vi "MessageCore.vi"(6 "Timeout (ms)":i32=-1, 8 "error in (no error)":errorcluster, 9 "Payload":string, 10 "Command":string, 11 "GRPCClient in":refnum<class "MicronTemplateAPIs.lvclass">) -> (0 "error out":errorcluster, 2 "Response":string, 3 "GRPCClient out":refnum<class "MicronTemplateAPIs.lvclass">)   [LabVIEW 2019, in "MicronTemplateAPIs.lvlib" / "MicronTemplateAPIs.lvclass"]
uses:
  MicronTemplateAPIs.lvclass
  vi.lib/Micron/gRPC/Client/MicronGRPCClient.lvclass
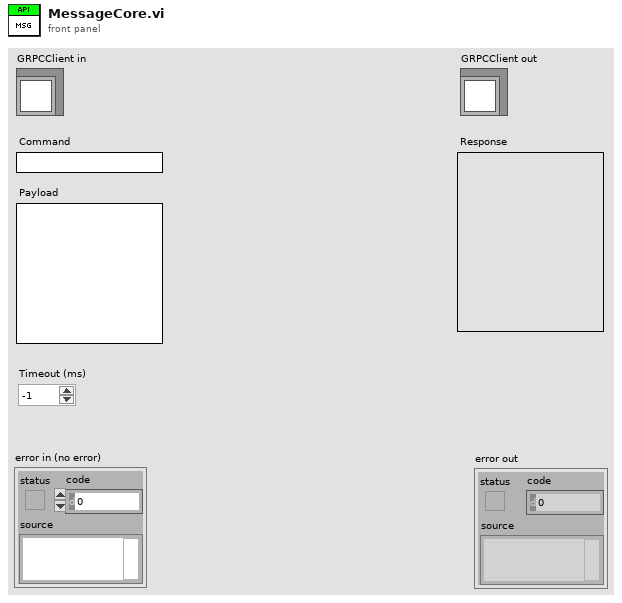
[diagram p1: front panel]
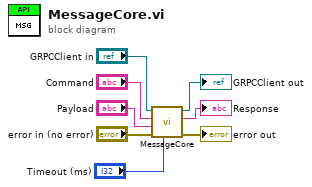
[diagram p0: block diagram]
diagram:
  n1 = call-parent "MessageCore.vi"("Timeout (ms)"="Timeout (ms)", "error in (no error)"="error in (no error)", "Payload"="Payload", "Command"="Command", "GRPCClient in"="GRPCClient in") -> ("error out"=→"error out":errorcluster, "Response"=→"Response":string, "GRPCClient out"=→"GRPCClient out":refnum<class "MicronTemplateAPIs.lvclass">)  [unwired: 4 in]
